vi "temp coef to color converter.vi"(2 "Temp Coef select":T1=enum."Red - 50 ppm/K") -> (6 "Temp Coef Color":u32(colorbox))   [LabVIEW 2018]
uses:
  temp coeficient--enum.ctl
  Resistor Band Colors/Resistor Band Colors.lvlib
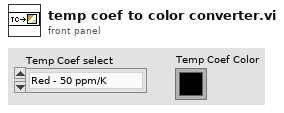
[diagram p1: front panel]
types:
  T1 = typedef "temp coeficient--enum.ctl" = enum16{"Grey - 1 ppm/K", "Violet - 5 ppm/K", "Blue - 10 ppm/K", "Green - 20 ppm/K", "Yellow - 25 ppm/K", "Orange - 15 ppm/K", "Red - 50 ppm/K", "Brown - 100 ppm/K", "Black - 250 ppm/K"}
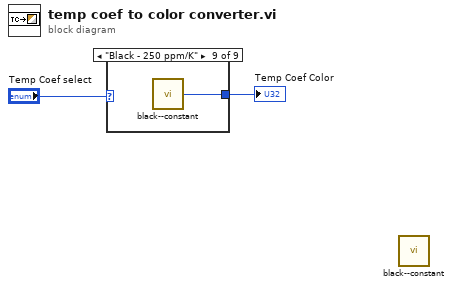
[diagram p0: block diagram]
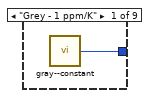
[diagram p2: hidden frame]
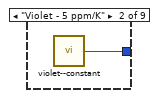
[diagram p3: hidden frame]
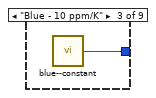
[diagram p4: hidden frame]
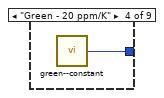
[diagram p5: hidden frame]
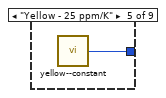
[diagram p6: hidden frame]
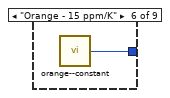
[diagram p7: hidden frame]
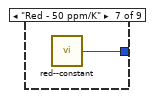
[diagram p8: hidden frame]
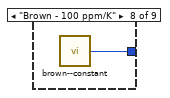
[diagram p9: hidden frame]
diagram:
  n1 = case shown="\"Black - 250 ppm/K\"" "Temp Coef select" {
    tunnel: [w3 w4 w5 w6 w7 w8 w9 w10 w11] -> w1
    frame "Grey - 1 ppm/K" {
      n2 = call "gray--constant.vi"() -> ("Gray"=w3:u32)  [unwired: 5 in]
    }
    frame "Violet - 5 ppm/K" {
      n3 = call "violet--constant.vi"() -> ("Violet"=w4:u32)  [unwired: 5 in]
    }
    frame "Blue - 10 ppm/K" {
      n4 = call "blue--constant.vi"() -> ("Blue"=w5:u32)  [unwired: 5 in]
    }
    frame "Green - 20 ppm/K" {
      n5 = call "green--constant.vi"() -> ("Green"=w6:u32)  [unwired: 5 in]
    }
    frame "Yellow - 25 ppm/K" {
      n6 = call "yellow--constant.vi"() -> ("Yellow"=w7:u32)  [unwired: 5 in]
    }
    frame "Orange - 15 ppm/K" {
      n7 = call "orange--constant.vi"() -> ("Orange"=w8:u32)  [unwired: 5 in]
    }
    frame "Red - 50 ppm/K" {
      n8 = call "red--constant.vi"() -> ("Red"=w9:u32)  [unwired: 5 in]
    }
    frame "Brown - 100 ppm/K" {
      n9 = call "brown--constant.vi"() -> ("Brown"=w10:u32)  [unwired: 5 in]
    }
    frame "Black - 250 ppm/K" {
      n10 = call "black--constant.vi"() -> ("Black"=w11:u32)  [unwired: 5 in]
    }
  }
  "Temp Coef Color" <- w1
  n11 = call "black--constant.vi"() -> ()  [unwired: 5 in, 1 out]
